vi "Buffer Operations.vi"(8 "error in (no error)":errorcluster, 9 "Buffer Label (\"Buffer\")":string="Buffer", 10 "Operation (Start Buffer)":i32(ring) items=["Start Buffer", "Stop Buffer", "Clear Buffer", "Delete Buffer", "Continue Buffer"], 11 "VISA resource name":refnum<visa-resource-name>) -> (0 "error out":errorcluster, 3 "VISA resource name out":refnum<visa-resource-name>)   [LabVIEW 2020, in "Rohde&Schwarz CMXP Base.lvlib"]
doc: "Creates and activates a buffer. If the buffer exists already, it is cleared (equivalent to CLEar:BASE:BUFFer).\n\nAttributes:\nRSCMXPBASE_ATTR_START_BUFFER\nRSCMXPBASE_ATTR_STOP_BUFFER\nRSCMXPBASE_ATTR_CLEAR_BUFFER\nRSCMXPBASE_ATTR_DELETE_BUFFER\nRSCMXPBASE_ATTR_CONTINUE_BUFFER\n\nRemote-control commands:\nSTARt:BASE:BUFFer\nSTOP:BASE:BUFFer\nCLEar:BASE:BUFFer\nDELete:BASE:BUFFer\nCONTinue:BASE:BUFFer"
uses:
  <instrlib>/Rohde&Schwarz CMXP Base/Rohde&Schwarz CMXP Base.lvlib
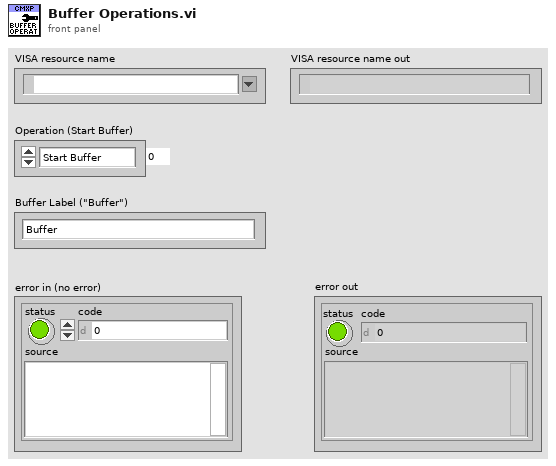
[diagram p1: front panel]
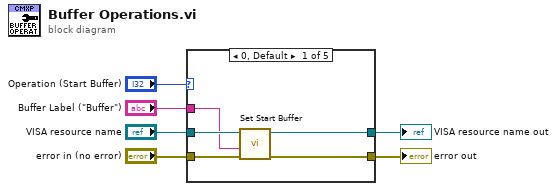
[diagram p0: block diagram]
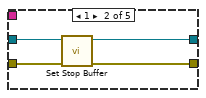
[diagram p2: hidden frame]
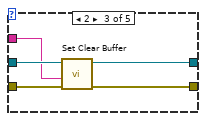
[diagram p3: hidden frame]
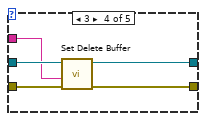
[diagram p4: hidden frame]
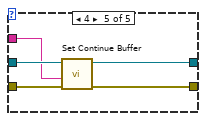
[diagram p5: hidden frame]
diagram:
  n1 = case shown="0, Default" "Operation (Start Buffer)" {
    tunnel: "error in (no error)" -> [w11 w15 w20 w25 w30]
    tunnel: "VISA resource name" -> [w10 w14 w19 w24 w29]
    tunnel: [w9 w13 w18 w23 w28] -> w4
    tunnel: [w8 w12 w17 w22 w27] -> w3
    tunnel: "Buffer Label (\"Buffer\")" -> [w7 _ w16 w21 w26]
    frame 0, Default {
      n2 = call "Set Start Buffer"("error in (no error)"=w11, "Start Buffer ()"=w7, "instrument handle"=w10) -> ("error out"=w9:errorcluster, "instrument handle out"=w8:refnum<visa-resource-name>)  [unwired: 7 in]
    }
    frame 1 {
      n3 = call "Set Stop Buffer"("error in (no error)"=w15, "instrument handle"=w14) -> ("error out"=w13:errorcluster, "instrument handle out"=w12:refnum<visa-resource-name>)  [unwired: 8 in]
    }
    frame 2 {
      n4 = call "Set Clear Buffer"("error in (no error)"=w20, "Clear Buffer ()"=w16, "instrument handle"=w19) -> ("error out"=w18:errorcluster, "instrument handle out"=w17:refnum<visa-resource-name>)  [unwired: 7 in]
    }
    frame 3 {
      n5 = call "Set Delete Buffer"("error in (no error)"=w25, "Delete Buffer ()"=w21, "instrument handle"=w24) -> ("error out"=w23:errorcluster, "instrument handle out"=w22:refnum<visa-resource-name>)  [unwired: 7 in]
    }
    frame 4 {
      n6 = call "Set Continue Buffer"("error in (no error)"=w30, "Continue Buffer ()"=w26, "instrument handle"=w29) -> ("error out"=w28:errorcluster, "instrument handle out"=w27:refnum<visa-resource-name>)  [unwired: 7 in]
    }
  }
  "error out" <- w4
  "VISA resource name out" <- w3
